vi "Lesen_verknuepfen.vi"(8 "error in (no error)":errorcluster caption="Fehler (Eingang, kein Fehler)", 9 "Order":string, 11 "param":string) -> (0 "error out":errorcluster caption="Fehler (Ausgang)", 3 "Verknüpfter String":string)   [LabVIEW 2020, in "Linearisierung v2.lvlib" / "Gasteiler.lvlib" / "HovaCAL_Interface.lvlib" / "KGN.lvlib"]
uses:
  KGN.lvlib
panel:
  in  "Zieladresse":string="FF"
  in  "Quelladresse":string="00"
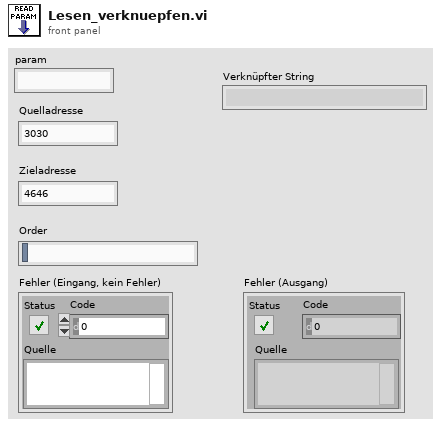
[diagram p1: front panel]
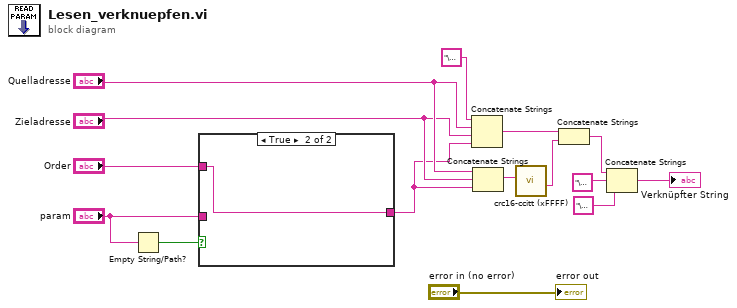
[diagram p0: block diagram]
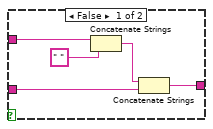
[diagram p2: hidden frame]
diagram:
  n1 = Empty String/Path?(string/path="param") -> (empty?=w1:bool)
  n2 = case shown="True" w1 {
    tunnel: "Order" -> [w20 w21]
    tunnel: [w19 w21] -> w4
    tunnel: "param" -> [w16 _]
    frame False {
      n3 = Concatenate Strings(w20, " " ("String")) -> (w18:string)
      n4 = Concatenate Strings(w18, w16) -> (w19:string)
    }
    frame True {
    }
  }
  n5 = Concatenate Strings("\u0002", "Quelladresse", "Zieladresse", w4) -> (w9:string)
  n6 = Concatenate Strings("Quelladresse", "Zieladresse", w4) -> (w7:string)
  n7 = call "crc16-ccitt (xFFFF).vi"("Message"=w7) -> ("Hex-Integer-String"=w6:string)  [unwired: 8 in, 2 out]
  n8 = Concatenate Strings(w9, w6) -> (w12:string)
  n9 = Concatenate Strings(w12, "\u0003", "\u0006" ("String")) -> (→"Verknüpfter String":string)
  "error out" <- "error in (no error)"
